vi "Read Description.vi"(9 "Page in":refnum<class "Page.lvclass">) -> (3 "Page out":refnum<class "Page.lvclass">, 4 "Description":string)   [LabVIEW 2014, in "Raspberry Pi Compatible Compiler for LabVIEW.lvlib" / "Page.lvclass"]
uses:
  Page.lvclass
  Page.lvclass/Page.ctl
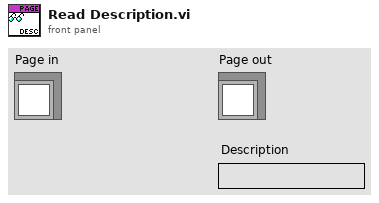
[diagram p1: front panel]
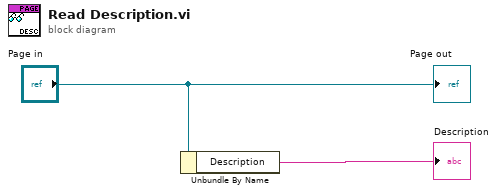
[diagram p0: block diagram]
diagram:
  n1 = Unbundle By Name("Page in") -> ("Description"=→"Description":string)
  "Page out" <- "Page in"
